vi "render_overlay_guides.vi"(6 "Guides":T1(array[cluster]), 7 "Image Out 2":T2) -> (3 "Image Out":T2)   [LabVIEW 2015]
uses:
  <vilib>/vision/Image Controls.llb/IMAQ Image.ctl
  red_tweezers_globals_INTERNAL.vi
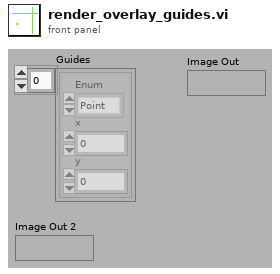
[diagram p1: front panel]
types:
  T1 = cluster{"Enum":enum16{"Point", "Cross", "Vertical", "Horizontal"}, "x":dbl, "y":dbl}[]
  T2 = typedef "IMAQ Image.ctl" = refnum<image>
  T3 = enum16{"Point", "Cross", "Vertical", "Horizontal"}
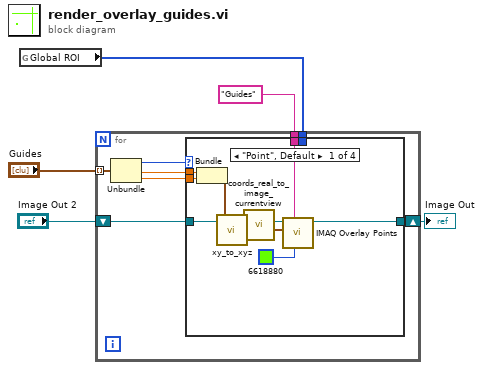
[diagram p0: block diagram]
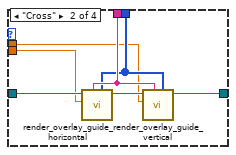
[diagram p2: hidden frame]
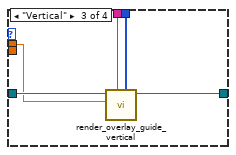
[diagram p3: hidden frame]
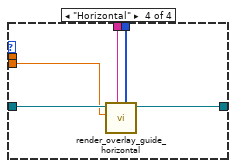
[diagram p4: hidden frame]
diagram:
  n1 = global read "red_tweezers_globals_INTERNAL.vi" "Global ROI"() -> (w1:i32[])
  n2 = for {
    tunnel: "Guides" -> [w13] mode=indexing
    shift-right: [w10] -> w5
    shift-left: "Image Out 2" -> [w11]
    tunnel: "Guides" ("Group") -> [w9]
    tunnel: w1 -> [w8]
    n3 = Unbundle(w13) -> ("Enum"=w12:T3, "x"=w7:dbl, "y"=w6:dbl)
    n4 = case shown="\"Point\", Default" w12 {
      tunnel: w11 -> [w22 w27 w32 w39]
      tunnel: [w21 w29 w31 w38] -> w10
      tunnel: w9 -> [w19 w26 w34 w37]
      tunnel: w8 -> [_ w25 w33 w36]
      tunnel: w7 -> [w17 w23 w30 _]
      tunnel: w6 -> [w16 w24 _ w35]
      frame "Point", Default {
        n5 = Bundle("x"=w17, "y"=w16) -> (w15:cluster{"x":dbl, "y":dbl})  [unwired: 1 in]
        n6 = call "xy_to_xyz.vi"("Position (2D)"=w15) -> ("Position (3D)"=w18:cluster{dbl, dbl, dbl})  [unwired: 3 in]
        n7 = call "coords_real_to_image_currentview.vi"("Position (real coords)"=w18) -> ("Position (pixels, relative to the top left of the image)"=w14:cluster{dbl, dbl})  [unwired: 7 in, 1 out]
        n8 = call "IMAQ Overlay Points"("Color"=u32 6618880, "Group"=w19, "Point"=w14, "Image"=w22) -> ("Image Out"=w21:T2)  [unwired: 6 in, 1 out]
      }
      frame "Cross" {
        n9 = call "render_overlay_guide_horizontal.vi"("ROI"=w25, "Group"=w26, "Position (real coords)"=w24, "Image"=w27) -> ("Image Out"=w28:T2)  [unwired: 5 in]
        n10 = call "render_overlay_guide_vertical.vi"("ROI"=w25, "Group"=w26, "Position (real coords)"=w23, "Image"=w28) -> ("Image Out"=w29:T2)  [unwired: 5 in]
      }
      frame "Vertical" {
        n11 = call "render_overlay_guide_vertical.vi"("ROI"=w33, "Group"=w34, "Position (real coords)"=w30, "Image"=w32) -> ("Image Out"=w31:T2)  [unwired: 5 in]
      }
      frame "Horizontal" {
        n12 = call "render_overlay_guide_horizontal.vi"("ROI"=w36, "Group"=w37, "Position (real coords)"=w35, "Image"=w39) -> ("Image Out"=w38:T2)  [unwired: 5 in]
      }
    }
  }
  "Image Out" <- w5
